vi "AD设置通道范围.vi"(8 "错误输入":errorcluster caption="错误输入（无错误）", 9 "起始通道":i32, 10 "终止通道":i32, 11 "设备句柄入":i32) -> (0 "错误输出":errorcluster, 3 "设备句柄":i32=1)   [LabVIEW 2016]
uses:
  dll/em9636.dll
panel:
  in  "超时毫秒":i32=1000
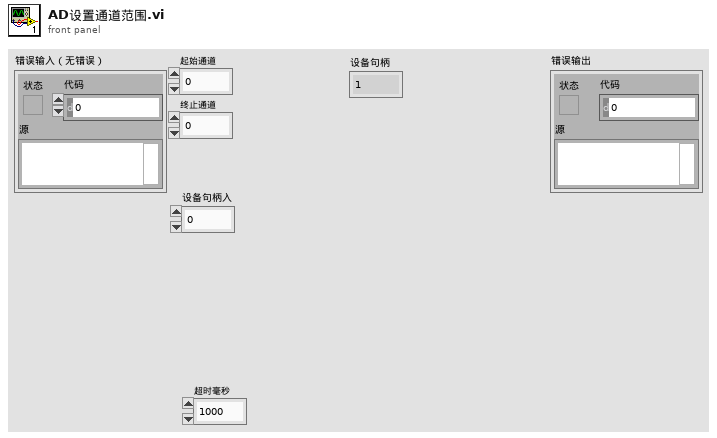
[diagram p1: front panel]
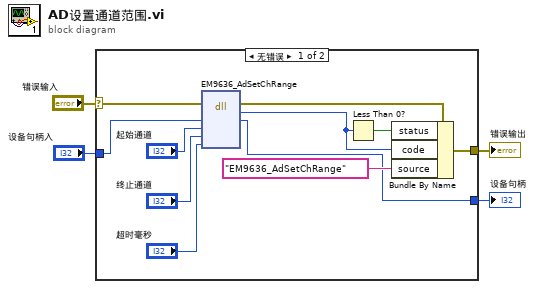
[diagram p0: block diagram]
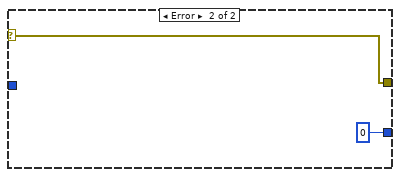
[diagram p2: hidden frame]
diagram:
  n1 = case shown="无错误" "错误输入" {
    selector: "错误输入" -> [w15 w17]
    tunnel: [w11 w17] -> w3
    tunnel: [w5 0 ("错误")] -> w2
    tunnel: "设备句柄入" -> [w9 _]
    frame No Error {
      n2 = dll-call lib="PTH2kabs CUsers\nAdministratorDesktopEM9636*EM9636系列_demo_labview(调用DLL方式)dll\nem9636.dll" fn="EM9636_AdSetChRange"(error in=w15, "设备句柄"=w9, "起始通道"="起始通道", "终止通道"="终止通道", "超时毫秒"="超时毫秒") -> (error out=w13:errorcluster, "错误"=w10:i32, "设备句柄"=w5:i32)  [unwired: 5 in, 1 out]
      n3 = Less Than 0?(x=w10) -> (x < 0?=w12:bool)
      n4 = Bundle By Name(cluster=w13, "status"=w12, "code"=w10, "source"="EM9636_AdSetChRange") -> (w11:errorcluster)
    }
    frame Error {
    }
  }
  "错误输出" <- w3
  "设备句柄" <- w2
